vi "Bin SGL Image.vi"(0 "Image Src":T1, 1 "X Binning":i32=1 min=1, 2 "Image Dst (SGL)":T1, 3 "error in (no error)":errorcluster, 5 "Y Binning":i32=1 min=1) -> (7 "Image Dst":T1, 9 "error out":errorcluster)   [LabVIEW 2021, in "Image.lvlib"]
uses:
  Image.lvlib
  <vilib>/vision/Image Controls.llb/IMAQ Image.ctl
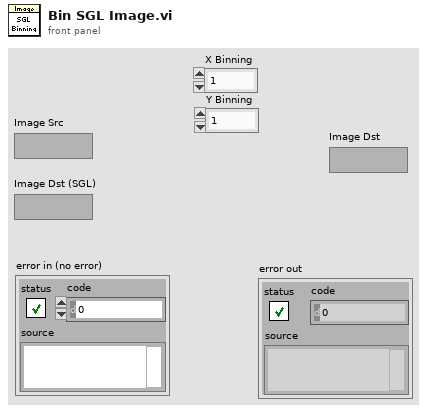
[diagram p1: front panel]
types:
  T1 = typedef "IMAQ Image.ctl" = refnum<image>
  T2 = typedef "Image Type" = u32
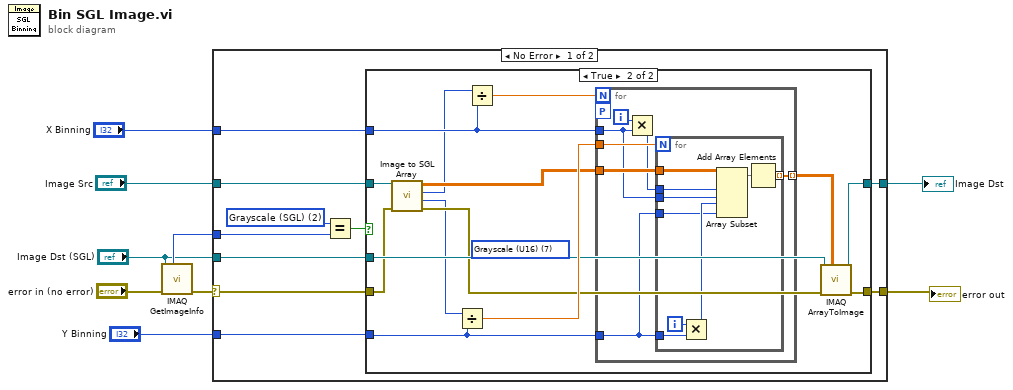
[diagram p0: block diagram]
diagram:
  n1 = call "IMAQ GetImageInfo"("error in (no error)"="error in (no error)", "Image"="Image Dst (SGL)") -> ("error out"=w9:errorcluster, "Image Type"=w8:T2)  [unwired: 2 in, 6 out]
  n2 = case shown="No Error" w9 {
    selector: w9 -> [w19 w53]
    tunnel: w8 -> [w17 _]
    tunnel: "Image Src" -> [w15 _]
    tunnel: [w14 w52] -> w6
    tunnel: [w13 w53] -> w4
    tunnel: "X Binning" -> [w12 _]
    tunnel: "Y Binning" -> [w11 _]
    tunnel: "Image Dst (SGL)" -> [w10 w52]
    frame No Error {
      w18 = T2 2 items=["Grayscale (U8)", "Grayscale (I16)", "Grayscale (SGL)", "Complex (CSG)", "RGB (U32)", "HSL (U32)", "RGB (U64)", "Grayscale (U16)"] ("Image Type")
      n3 = Equal?(x=w18, y=w17) -> (x = y?=w16:bool)
      n4 = case shown="True" w16 {
        tunnel: w19 -> [w20 w26]
        tunnel: w15 -> [w21 w27]
        tunnel: [w21 w28] -> w14
        tunnel: [w20 w29] -> w13
        tunnel: w12 -> [_ w33]
        tunnel: w11 -> [_ w32]
        tunnel: w10 -> [_ w30]
        frame False {
        }
        frame True {
          (unwired) T2 7 items=["Grayscale (U8)", "Grayscale (I16)", "Grayscale (SGL)", "Complex (CSG)", "RGB (U32)", "HSL (U32)", "RGB (U64)", "Grayscale (U16)"] ("Image Type")
          n5 = call "Image to SGL Array.vi"("error in (no error)"=w26, "Image"=w27) -> ("error out"=w25:errorcluster, "Y Resolution"=w22:i32, "X Resolution"=w23:i32, "Image Pixels (Float)"=w24:sgl[][])  [unwired: 6 in]
          n6 = Divide(x=w22, y=w32) -> (x/y=w34:dbl)
          n7 = Divide(x=w23, y=w33) -> (x/y=w35:dbl)
          n8 = for {
            N: w35 -> [_]
            tunnel: w24 -> [w42]
            tunnel: w34 -> [w41]
            tunnel: w33 -> [w38]
            tunnel: w32 -> [w37]
            tunnel: [w36] -> w31 mode=indexing
            workers-P: _ -> [_]
            i -> [w40]
            n9 = Multiply(x=w40, y=w38) -> (x*y=w39:i32)
            n10 = for {
              N: w41 -> [_]
              tunnel: w42 -> [w49]
              tunnel: w37 -> [w50]
              tunnel: w39 -> [w48]
              tunnel: w38 -> [w46]
              tunnel: w37 -> [w45]
              tunnel: [w43] -> w36 mode=indexing
              i -> [w51]
              n11 = Multiply(x=w51, y=w50) -> (x*y=w47:i32)
              n12 = Array Subset(array=w49, index (row)=w48, length (row)=w46, index (col)=w47, length (col)=w45) -> (w44:sgl[][])
              n13 = Add Array Elements(numeric array=w44) -> (sum=w43:sgl)
            }
          }
          n14 = call "IMAQ ArrayToImage"("Image Pixels (Float)"=w31, "error in (no error)"=w25, "Image"=w30) -> ("error out"=w29:errorcluster, "Image Out"=w28:T1)  [unwired: 7 in]
        }
      }
    }
    frame Error {
    }
  }
  "error out" <- w4
  "Image Dst" <- w6
